vi "AutoScaleGraph.vi"(1 "Array":dbl[](array[numeric]), 2 "WaveformGraph in":refnum<vi>) -> ()   [LabVIEW 2014]
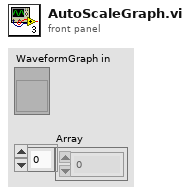
[diagram p1: front panel]
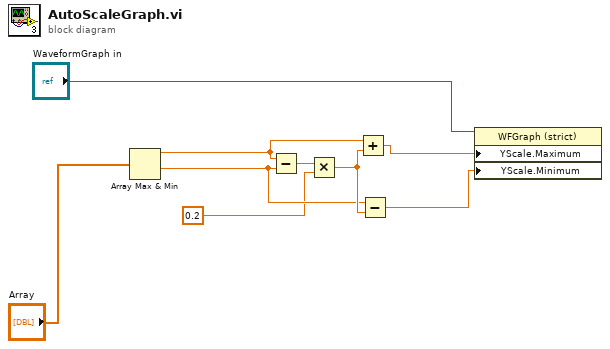
[diagram p0: block diagram]
diagram:
  n1 = Array Max & Min(array="Array") -> (max value=w4:dbl, min value=w5:dbl)  [unwired: 2 out]
  n2 = Subtract(x=w4, y=w5) -> (x-y=w2:dbl)
  n3 = Multiply(x=w2, y=0.2) -> (x*y=w6:dbl)
  n4 = Add(x=w4, y=w6) -> (x+y=w7:dbl)
  n5 = Subtract(x=w5, y=w6) -> (x-y=w8:dbl)
  n6 = property on="Property Node" class="WFGraph (strict)"(reference="WaveformGraph in", "YScale.Maximum"=w7, "YScale.Minimum"=w8) -> ()  [unwired: 1 in, 2 out]
